vi "Mean Time to Acknowledged.vi"(8 "error in (no error)":errorcluster, 11 "alarms in":refnum<class "NI SystemLink Alarm.lvclass">[](array[class])) -> (0 "error out":errorcluster, 1 "MTTA of alarms (days)":dbl format="%#.2g", 2 "MTTA of alarms (HH:MM:SS)":dbl format="%<%H:%M:%S>t", 3 "alarms out":refnum<class "NI SystemLink Alarm.lvclass">[](array[class]), 4 "MTTA Array":dbl[](array[numeric]) format="%<%H:%M:%S>t", 5 "# of acknowledged alarms":i32)   [LabVIEW 2019, in "SystemLink Alarm KPIs.lvlib"]
uses:
  SystemLink Alarm KPIs.lvlib
  <vilib>/Skyline/Alarm/Class/NI SystemLink Alarm.lvclass
  <vilib>/Skyline/Alarm/Class/NI SystemLink Alarm.lvclass/NI SystemLink Alarm.ctl
  <vilib>/Skyline/Alarm/Class/Accessors/Read Acknowledged At.vi
  <vilib>/Skyline/Alarm/Class/Accessors/Read Acknowledged.vi
  <vilib>/Analysis/baseanly.llb/Mean (DBL).vi
  <vilib>/Skyline/Alarm/Class/Private/Ensure Alarm Information.vi
  <vilib>/Skyline/Alarm/Class/Accessors/Read Transitions.vi
  <vilib>/Skyline/Alarm/Library/Get Alarm Information.vi
  <vilib>/Analysis/NI_AALBase.lvlib
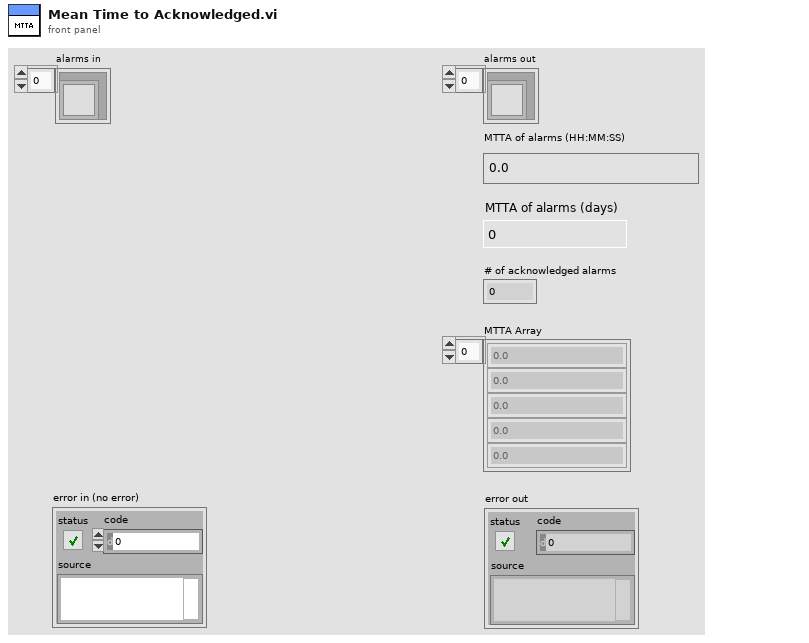
[diagram p1: front panel]
types:
  T1 = typedef "NI SystemLink Alarm Library.lvlib/Transition.ctl" = cluster{"type":T2, "severity level":T3, "condition":string, "occurred at":timestamp, "keywords":string[], "properties":T4[]}
  T2 = typedef "NI SystemLink Alarm Library.lvlib/Transition Type.ctl" = enum16{"Set", "Clear"}
  T3 = typedef "NI SystemLink Alarm Library.lvlib/Severity Level.ctl" = i32
  T4 = typedef "NI Skyline Utilities.lvlib/Property.ctl" = cluster{"key":string, "value":string}
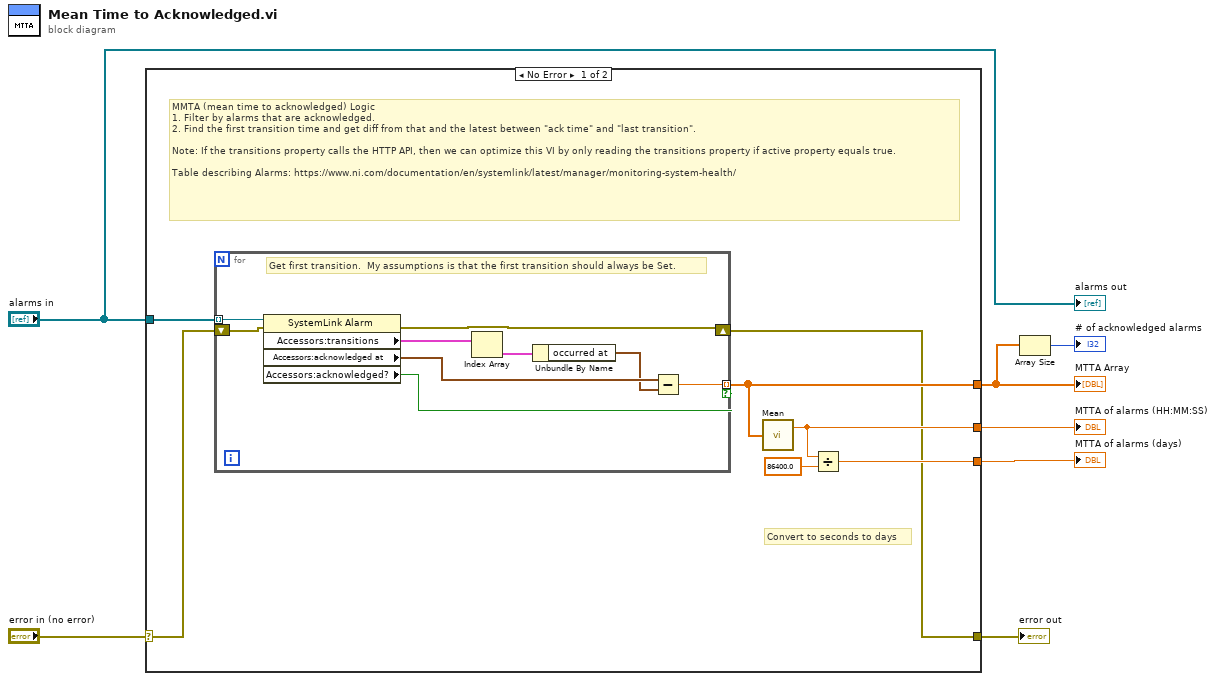
[diagram p0: block diagram]
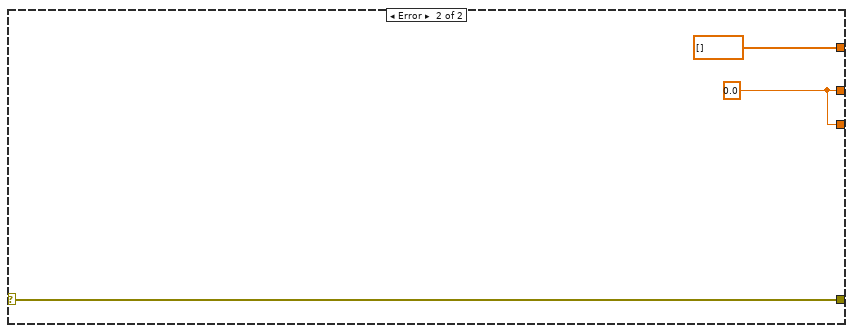
[diagram p2: hidden frame]
diagram:
  n1 = case shown="No Error" "error in (no error)" {
    selector: "error in (no error)" -> [w9 w24]
    tunnel: [w14 dbl[] []] -> w2
    tunnel: [w12 w25] -> w7
    tunnel: "alarms in" -> [w11 _]
    tunnel: [w10 w25] -> w5
    tunnel: [w8 w24] -> w3
    frame No Error {
      # "Convert to seconds to days"
      # "MMTA (mean time to acknowledged) Logic\n1. Filter by alarms that are acknowledged.\n2. Find the first transition time and get diff from that and the latest between \"ack time\" and \"last transition\".\n\nNote: If the transitions property calls the HTTP API, then we can optimize this VI by only reading the transitions property if active property equals true.\n\nTable describing Alarms: https://www.ni.com/documentation/en/systemlink/latest/manager/monitoring-system-health/"
      n2 = for {
        tunnel: w11 -> [w23] mode=indexing
        tunnel: [w18] -> w14 mode=indexing if=w15
        shift-right: [w16] -> w8
        shift-left: w9 -> [w17]
        # "Get first transition.  My assumptions is that the first transition should always be Set."
        n3 = property class="SystemLink Alarm"(reference=w23, error in=w17) -> (error out=w16:errorcluster, "Accessors:transitions"=w22:T1[], "Accessors:acknowledged at"=w20:timestamp, "Accessors:acknowledged?"=w15:bool)  [unwired: 1 out]
        n4 = Index Array(array=w22) -> (element=w21:T1)  [unwired: 1 in]
        n5 = Unbundle By Name(w21) -> ("occurred at"=w19:timestamp)
        n6 = Subtract(x=w20, y=w19) -> (x-y=w18:dbl)
      }
      n7 = call-poly <vilib>:"Mean.vi"("X"=w14) -> ("mean"=w10:dbl)  [unwired: 1 out]
      n8 = Divide(x=w10, y=86400.0) -> (x/y=w12:dbl)
    }
    frame Error {
      w25 = 0.0 ("mean")
    }
  }
  "MTTA Array" <- w2
  "MTTA of alarms (HH:MM:SS)" <- w5
  "MTTA of alarms (days)" <- w7
  "error out" <- w3
  n9 = Array Size(array=w2) -> (size(s)=→"# of acknowledged alarms":i32)
  "alarms out" <- "alarms in"
